vi "Get Unique Test ID.vi"(1 "Elite DAQ Board in":refnum<class "Elite DAQ Design.lvclass">) -> (0 "id #":u32)   [LabVIEW 2023, in "Elite DAQ Design.lvclass"]
doc: "Get an identification number."
uses:
  Elite DAQ Design.lvclass
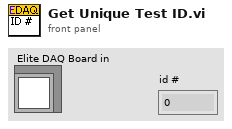
[diagram p1: front panel]
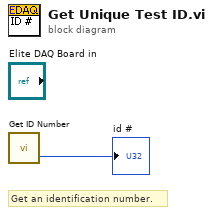
[diagram p0: block diagram]
diagram:
  # "Get an identification number."
  n1 = call "Get ID Number.vi"() -> ("id number"=→"id #":u32)  [unwired: 2 in]
